vi "Test5.vi"() -> ()   [LabVIEW 2017]
panel:
  in  "CSelect":i32=33
  in  "TrxVal":i32=33
  out "OutVal":i32
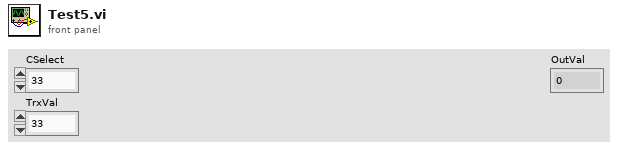
[diagram p1: front panel]
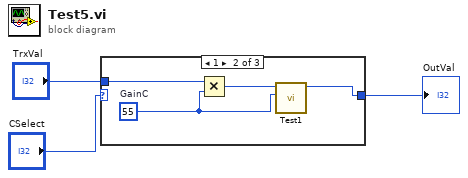
[diagram p0: block diagram]
diagram:
  n1 = case shown="1" "CSelect" {
    selector: "CSelect" -> [_ _ w9]
    tunnel: "TrxVal" -> [w4 w8 _]
    tunnel: [w4 w5 w9] -> w3
    frame 0, Default {
    }
    frame 1 {
      w7 = 55  # GainC
      n2 = Multiply(x=w8, y=w7) -> (x*y=w6:i32)
      n3 = call "Test1.vi"("B"=w7, "A"=w6) -> ("C"=w5:i32)  [unwired: 8 in, 1 out]
    }
    frame 2 {
    }
  }
  "OutVal" <- w3
